vi "rpr - optimal subspace.vi"(7 "dimension":i32=2, 9 "Array of peaks IN":dbl[][](array[numeric]), 10 "temperature points":dbl[](array[numeric]), 11 "peaks":i32[](array[numeric])) -> (0 "Array":dbl[][](array[numeric]), 1 "Array of clasters":cluster{"temperature points OUT":dbl[], dbl[]}[](array[cluster]), 2 "Array of clasters derivative":cluster{"temperature points OUT":dbl[], dbl[]}[](array[cluster]), 3 "Array of eigenvalues":dbl[](array[numeric]))   [LabVIEW 2014]
uses:
  <vilib>/Analysis/7linalg.llb/Eigenvalue and Vectors Output Option.ctl
  <vilib>/Analysis/_algsub.llb/Vector Norm Type.ctl
  <vilib>/Analysis/baseanly.llb/Real A x B.vi
  <vilib>/Analysis/_algsub.llb/Real Vector Norm.vi
  <vilib>/Analysis/Matrix/Numeric/Conversions/Array To Matrix - RA2.vi
  <vilib>/Analysis/7linalg.llb/Real Eigenvalues and Vectors.vi
  <vilib>/Analysis/Matrix/Numeric/Conversions/Matrix To Array - CM.vi
  <vilib>/Analysis/Matrix/NI_Matrix.lvlib
  <vilib>/Analysis/NI_AALPro.lvlib
  <vilib>/Analysis/NI_AALBase.lvlib
panel:
  out "number of columns":i32
  out "number of rows":i32
  out "sorted array":dbl[](array[numeric])
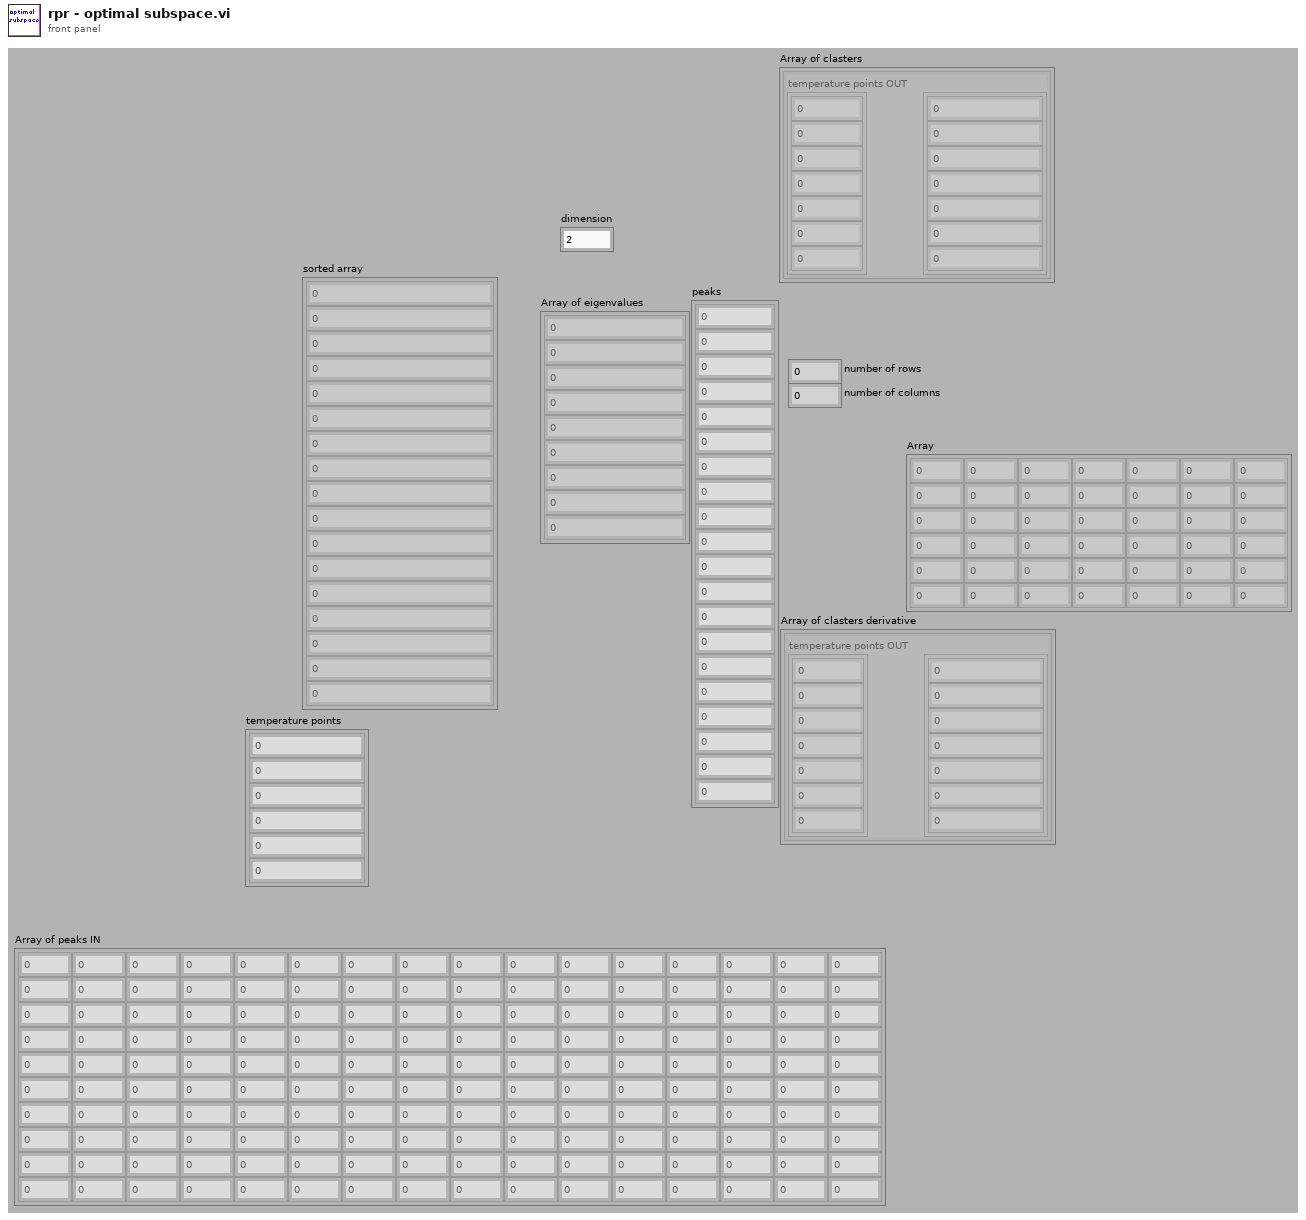
[diagram p1: front panel]
types:
  T1 = typedef "NI_AALPro.lvlib/Eigenvalue and Vectors Output Option.ctl" = i32
  T2 = typedef "NI_Matrix.lvlib/RealMatrix.ctl" = dbl[][]
  T3 = typedef "NI_Matrix.lvlib/ComplexMatrix.ctl" = cdb[][]
  T4 = typedef "NI_AALPro.lvlib/Vector Norm Type.ctl" = u16
  T5 = cluster{"temperature points":dbl[], "derivative (kHz/min)":dbl[]}
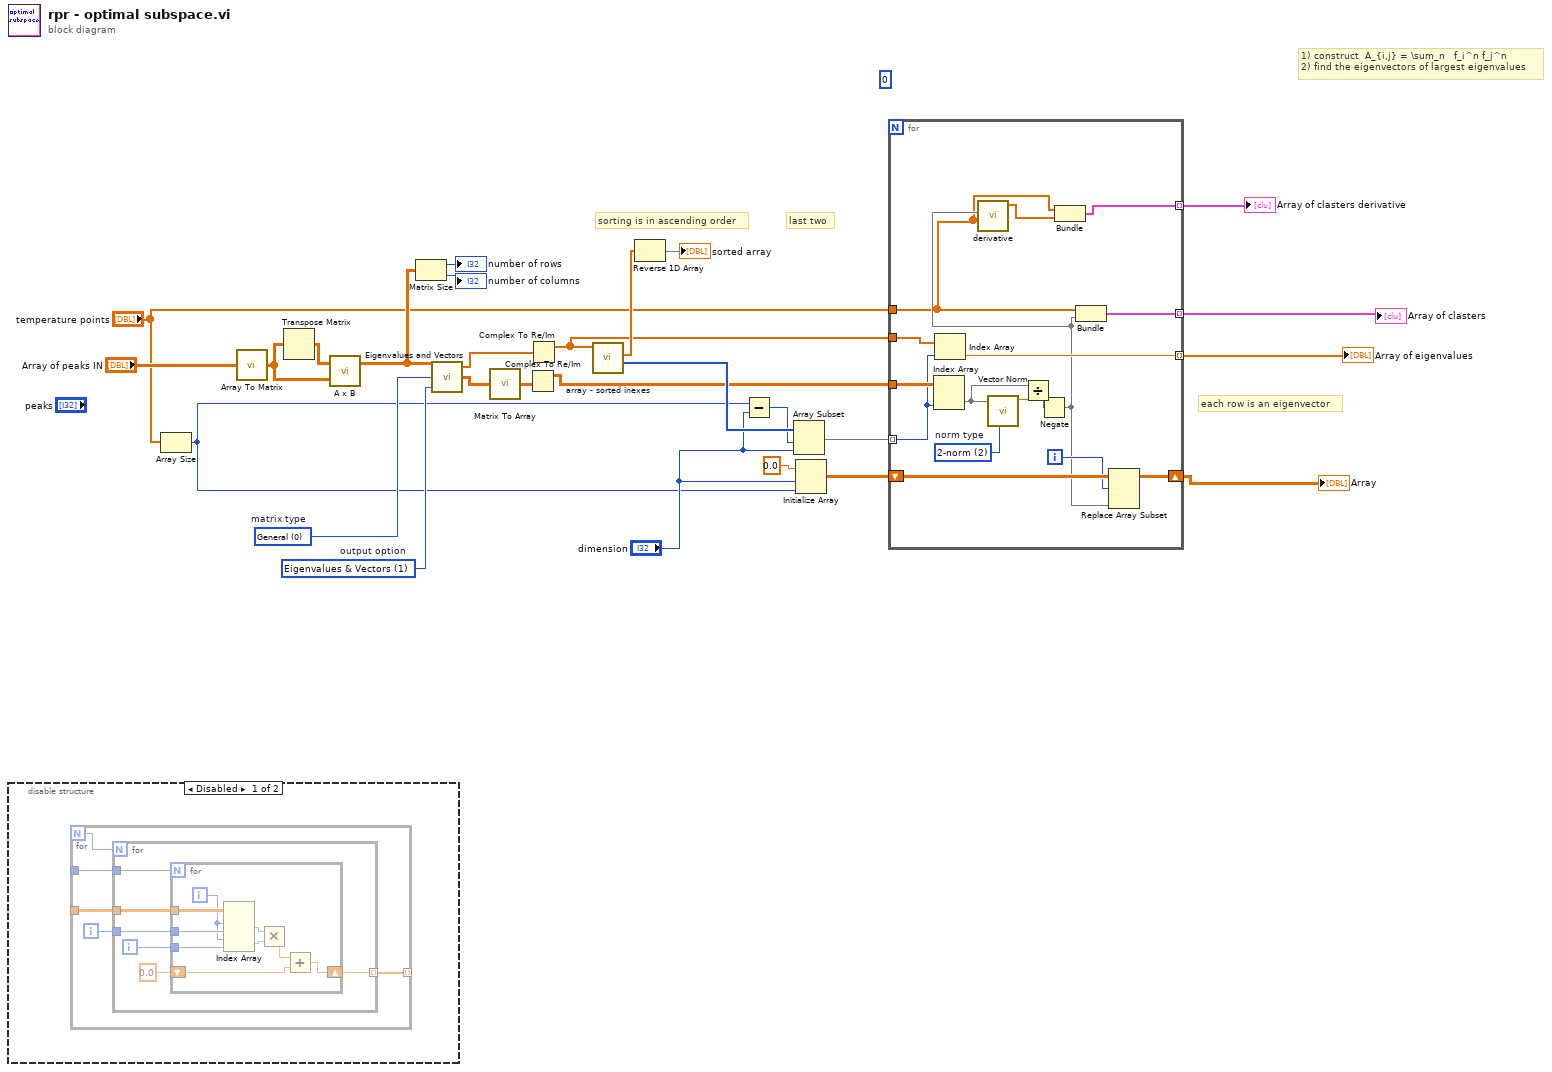
[diagram p0: block diagram]
diagram:
  (unwired) 0
  w24 = T1 1 items=["Eigenvalues", "Eigenvalues & Vectors"]  # output option
  w25 = 0 items=["General", "Symmetric"]  # matrix type
  # "1) construct  A_{i,j} = \\sum_n   f_i^n f_j^n \n2) find the eigenvectors of largest eigenvalues"
  # "sorting is in ascending order"
  # "last two"
  # "each row is an eigenvector"
  n1 = disable-structure shown="Disabled" {
    frame Disabled {
      n2 = for {
        N -> [w28]
        tunnel: _ -> [w32]
        tunnel: [w30] -> _ mode=indexing
        tunnel: _ -> [w29]
        i -> [w31]
        n3 = for {
          N: w28 -> [_]
          tunnel: w32 -> [w38]
          tunnel: w31 -> [w36]
          tunnel: [w34] -> w30 mode=indexing
          tunnel: w29 -> [w33]
          i -> [w37]
          n4 = for {
            N: w33 -> [_]
            tunnel: w38 -> [w47]
            tunnel: w37 -> [w46]
            tunnel: w36 -> [w45]
            shift-right: [w39] -> w34
            shift-left: 0.0 ("element") -> [w40]
            i -> [w44]
            n5 = Index Array(array=w47, index (row) #1=w44, index (col) #1=w45, index (row) #2=w44, index (col) #2=w46) -> (element #1=w43, element #2=w42)
            n6 = Multiply(x=w43, y=w42) -> (x*y=w41:dbl)
            n7 = Add(x=w41, y=w40) -> (x+y=w39:dbl)
          }
        }
      }
    }
    frame Enabled {
    }
  }
  n8 = Array Size(array="temperature points") -> (size(s)=w3:i32)
  n9 = call-poly <vilib>:"Array To Matrix.vi"("Real 2D Array"="Array of peaks IN") -> ("Real Matrix"=w9:T2)
  n10 = Transpose Matrix(1:w9) -> (0:w10:T2)
  n11 = call-poly <vilib>:"A x B.vi"("B"=w9, "A"=w10) -> ("A x B"=w8:T2)  [unwired: 1 out]
  n12 = Matrix Size(0:w8) -> (1:→"number of rows":i32, 2:→"number of columns":i32)
  n13 = call-poly <vilib>:"Eigenvalues and Vectors.vi"("output option"=w24, "matrix type"=w25, "Input Matrix"=w8) -> ("Eigenvectors"=w23:T3, "Eigenvalues"=w16:cdb[])  [unwired: 1 out]
  n14 = call-poly <vilib>:"Matrix To Array.vi"("Complex Matrix"=w23) -> ("Complex 2D Array"=w12:cdb[][])
  n15 = Complex To Re/Im(x + iy=w12) -> (x=w11:dbl[][])  [unwired: 1 out]
  n16 = Complex To Re/Im(x + iy=w16) -> (x=w5:dbl[])  [unwired: 1 out]
  n17 = call "array - sorted inexes.vi"("x"=w5) -> ("index array"=w22:i32[], "sorted array"=w14:dbl[])  [unwired: 9 in]
  n18 = Reverse 1D Array(array=w14) -> (reversed array=→"sorted array":dbl[])
  n19 = Subtract(x=w3, y="dimension") -> (x-y=w17:i32)
  n20 = Array Subset(array=w22, index=w17, length="dimension") -> (w21:i32[])
  n21 = Initialize Array(0.0 ("element"), "dimension", w3) -> (w19:dbl[][])
  n22 = for {
    tunnel: w11 -> [w63]
    tunnel: w21 -> [w57] mode=indexing
    shift-right: [w60] -> w27
    shift-left: w19 -> [w62]
    tunnel: "temperature points" -> [w49]
    tunnel: [w59] -> w26 mode=indexing
    tunnel: [w58] -> w15 mode=indexing
    tunnel: w5 -> [w56]
    tunnel: [w48] -> w1 mode=indexing
    i -> [w61]
    w55 = T4 2 items=["1-norm"=1, "2-norm"=2, "Inf-norm"=3, "-Inf-norm"=4, "User Defined"=5]  # norm type
    n23 = Index Array(array=w63, index (col)=w57) -> (element=w53:dbl[])  [unwired: 1 in]
    n24 = Index Array(array=w56, index=w57) -> (element=w58:dbl)
    n25 = call-poly <vilib>:"Vector Norm.vi"("norm type"=w55, "Input Vector"=w53) -> ("norm"=w54:dbl)  [unwired: 8 in, 1 out]
    n26 = Divide(x=w53, y=w54) -> (x/y=w52:dbl[])
    n27 = Negate(x=w52) -> (-x=w51:dbl[])
    n28 = call "derivative.vi"("temperature (min)"=w49, "frequency (kHz)"=w51) -> ("derivative (kHz/min)"=w50:dbl[])  [unwired: 9 in]
    n29 = Bundle("temperature points"=w49, "derivative (kHz/min)"=w50) -> (w48:T5)  [unwired: 1 in]
    n30 = Bundle("temperature points"=w49, w51) -> (w59:cluster{"temperature points":dbl[], dbl[]})  [unwired: 1 in]
    n31 = Replace Array Subset(array=w62, new element=w51, index (row)=w61) -> (w60:dbl[][])  [unwired: 1 in]
  }
  "Array" <- w27
  "Array of clasters" <- w26
  "Array of eigenvalues" <- w15
  "Array of clasters derivative" <- w1
